vi "uart_test1.vi"() -> ()   [LabVIEW 2020]
uses:
  <vilib>/Instr/_visa.llb/VISA Configure Serial Port (Instr).vi
panel:
  out "x/y 2":dbl
  out "x/y":dbl
  out "unsigned byte array":u8[](array[numeric])
  out "return count":u32
  in  "VISA resource name":refnum<visa-resource-name>
  in  "stop":bool
  out "x+y":dbl
  out "read buffer":string
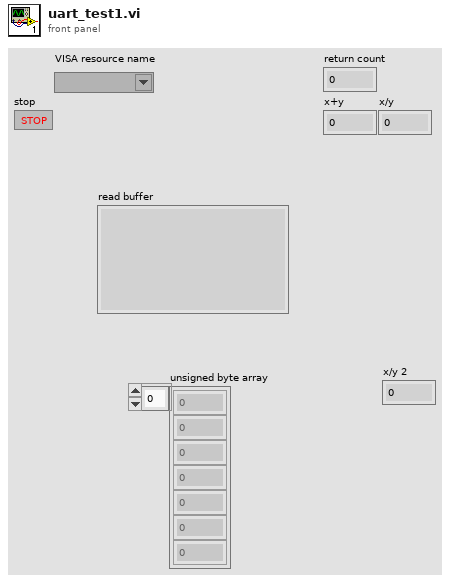
[diagram p1: front panel]
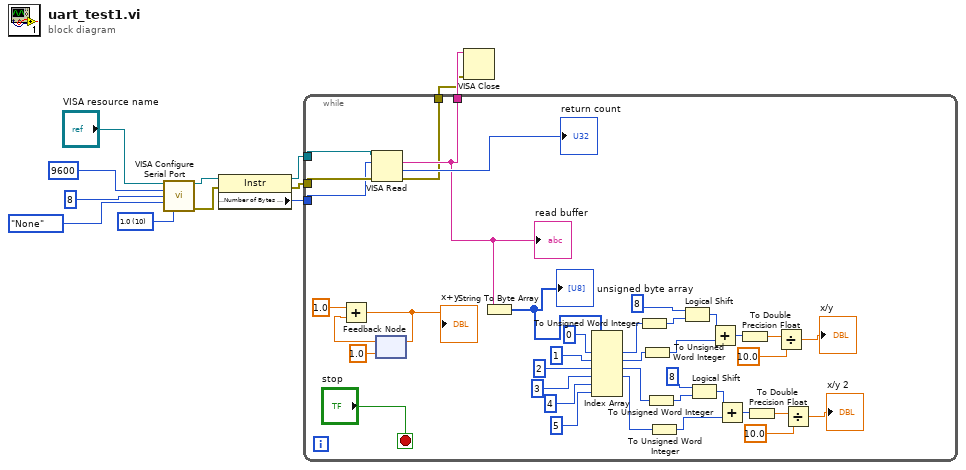
[diagram p0: block diagram]
diagram:
  w8 = u16 10 items=["1.0"=10, "1.5"=15, "2.0"=20] ("stop bits (10: 1 bit)")
  n1 = call-poly "VISA Configure Serial Port"("VISA resource name"="VISA resource name", "baud rate (9600)"=u32 9600, "data bits (8)"=u16 8, "parity (0:none)"=enum16{"None", "Odd", "Even", "Mark", "Space"}."None", "stop bits (10: 1 bit)"=w8) -> ("VISA resource name out"=w7:refnum<visa-resource-name>, "error out"=w6:errorcluster)  [unwired: 9 in]
  n2 = property class="Instr"(reference=w7, error in=w6) -> (reference out=w5:refnum<visa-resource-name>, error out=w4:errorcluster, "Serial Settings:Number of Bytes at Serial Port"=w3:u32)
  n3 = while {
    tunnel: w5 -> [w45]
    tunnel: w4 -> [w44]
    tunnel: w3 -> [w43]
    tunnel: [w34] -> w2
    tunnel: [w33] -> w1
    stop <- "stop" stop-if-true
    n4 = VISA Read(VISA resource name=w45, byte count=w43, error in (no error)=w44) -> (read buffer=w34:string, return count=→"return count":u32, error out=w33:errorcluster)  [unwired: 1 out]
    "read buffer" <- w34
    n5 = feedback #1(1.0) -> (w48:dbl)
    n6 = Add(x=1.0, y=w48) -> (x+y=w49:dbl)
    "x+y" <- w49
    n7 = feedback-in #1(w49) -> ()
    n8 = String To Byte Array(string=w34) -> (unsigned byte array=w41:u8[])
    "unsigned byte array" <- w41
    n9 = Index Array(array=w41, index #1=0 ("index"), index #2=1 ("index"), index #3=2 ("index"), index #4=3 ("index"), index #5=4 ("index"), index #6=5 ("index")) -> (element #1=w31:u8, element #2=w28:u8, element #3=w14:u8, element #4=w13:u8)  [unwired: 2 out]
    n10 = To Unsigned Word Integer(number=w31) -> (unsigned 16bit integer=w30:u16)
    n11 = To Unsigned Word Integer(number=w28) -> (unsigned 16bit integer=w27:u16)
    n12 = To Unsigned Word Integer(number=w14) -> (unsigned 16bit integer=w21:u16)
    n13 = To Unsigned Word Integer(number=w13) -> (unsigned 16bit integer=w19:u16)
    n14 = Logical Shift(y=u8 8 ("x"), x=w30) -> (x << y=w29:u16)
    n15 = Logical Shift(y=u8 8 ("x"), x=w21) -> (x << y=w20:u16)
    n16 = Add(x=w29, y=w27) -> (x+y=w26:u16)
    n17 = Add(x=w20, y=w19) -> (x+y=w18:u16)
    n18 = To Double Precision Float(number=w26) -> (double precision float=w25:dbl)
    n19 = To Double Precision Float(number=w18) -> (double precision float=w17:dbl)
    n20 = Divide(x=w25, y=10.0) -> (x/y=→"x/y":dbl)
    n21 = Divide(x=w17, y=10.0) -> (x/y=→"x/y 2":dbl)
  }
  n22 = VISA Close(VISA resource name=w2, error in (no error)=w1) -> ()  [unwired: 1 out]
